vi "字符串精度转换.vi"(7 "枚举":enum16{"小数位修约", "保留原始长度"}(ring), 9 "数组输入":string[](array[string]), 10 "数据精度":i32=6, 11 "输入字符串":string) -> (1 "数组输出":string[](array[string]), 3 "输出字符串":string)   [LabVIEW 2016, in "数据传输系统-05.lvlib"]
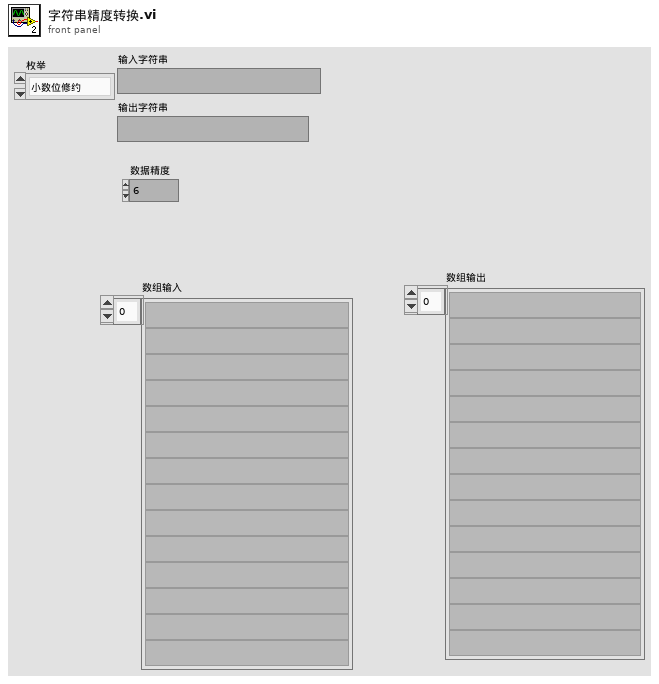
[diagram p1: front panel]
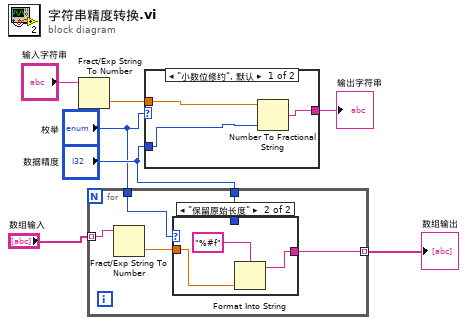
[diagram p0: block diagram]
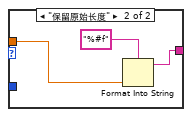
[diagram p2: hidden frame]
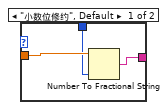
[diagram p3: hidden frame]
diagram:
  n1 = Fract/Exp String To Number(string="输入字符串") -> (number=w3:dbl)  [unwired: 3 in, 1 out]
  n2 = for {
    tunnel: "数组输入" -> [w11] mode=indexing
    tunnel: [w10] -> w4 mode=indexing
    tunnel: "数据精度" -> [w9]
    tunnel: "枚举" -> [w8]
    n3 = Fract/Exp String To Number(string=w11) -> (number=w12:dbl)  [unwired: 3 in, 1 out]
    n4 = case shown="\"保留原始长度\"" w8 {
      tunnel: w12 -> [w15 w16]
      tunnel: [w14 w17] -> w10
      tunnel: w9 -> [w13 _]
      frame "小数位修约", Default {
        n5 = Number To Fractional String(number=w15, precision (6)=w13) -> (F-format string=w14:string)  [unwired: 2 in]
      }
      frame "保留原始长度" {
        n6 = Format Into String(format string="%#f" ("格式字符串"), w16) -> (resulting string=w17:string)  [unwired: 2 in, 1 out]
      }
    }
  }
  "数组输出" <- w4
  n7 = case shown="\"小数位修约\", 默认" "枚举" {
    tunnel: [w21 w22] -> w6
    tunnel: w3 -> [w20 w23]
    tunnel: "数据精度" -> [w19 _]
    frame "小数位修约", Default {
      n8 = Number To Fractional String(number=w20, precision (6)=w19) -> (F-format string=w21:string)  [unwired: 2 in]
    }
    frame "保留原始长度" {
      n9 = Format Into String(format string="%#f" ("格式字符串"), w23) -> (resulting string=w22:string)  [unwired: 2 in, 1 out]
    }
  }
  "输出字符串" <- w6
